vi "getDecay.vi"(8 "error in (no error)":errorcluster, 11 "LaguerreDeconClass in":refnum<class "LaguerreDeconEngineClass.lvclass">) -> (0 "error out":errorcluster, 2 "Decay":dbl[](array[numeric]), 3 "LaguerreDeconClass out":refnum<class "LaguerreDeconEngineClass.lvclass">)   [LabVIEW 2020, in "LaguerreDeconEngineClass.lvclass"]
uses:
  LaguerreDeconEngineClass.lvclass
  LaguerreDeconEngineClass.lvclass/LaguerreDeconEngineClass.ctl
  <vilib>/Analysis/baseanly.llb/A x Vector.vi
  <vilib>/Analysis/NI_AALBase.lvlib
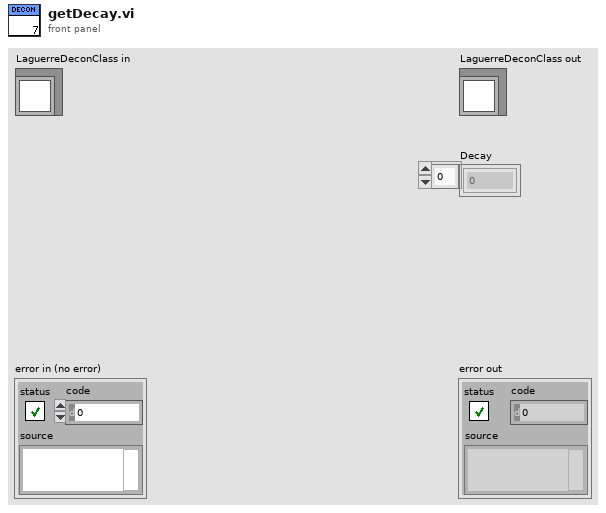
[diagram p1: front panel]
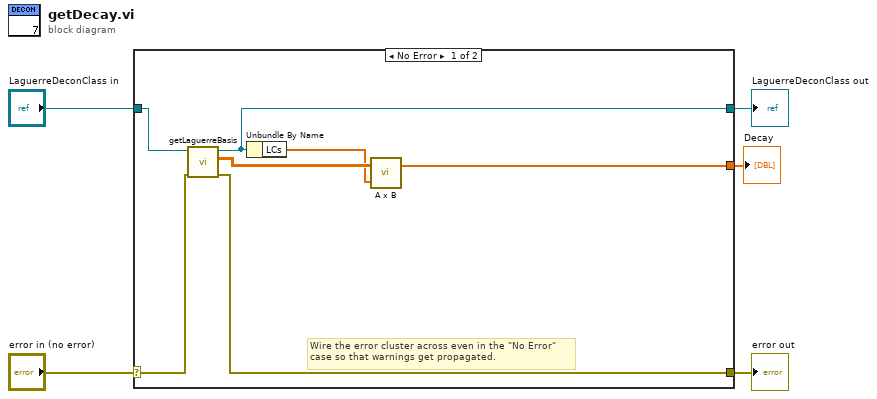
[diagram p0: block diagram]
diagram:
  n1 = case shown="No Error" "error in (no error)" {
    selector: "error in (no error)" -> [w9 w14]
    tunnel: [w8 w14] -> w4
    tunnel: [w6 w13] -> w2
    tunnel: "LaguerreDeconClass in" -> [w12 w13]
    tunnel: [w7 _] -> w1
    frame No Error {
      # "Wire the error cluster across even in the \"No Error\"\ncase so that warnings get propagated."
      n2 = call "getLaguerreBasis.vi"("error in (no error)"=w9, "LaguerreDeconClass in"=w12) -> ("error out"=w8:errorcluster, "laguerreBasis"=w11:dbl[][], "LaguerreDeconClass out"=w6:refnum<class "LaguerreDeconEngineClass.lvclass">)  [unwired: 7 in]
      n3 = Unbundle By Name(w6) -> ("LCs"=w10:dbl[])
      n4 = call-poly <vilib>:"A x B.vi"("Vector"=w10, "A"=w11) -> ("A x Vector"=w7:dbl[])  [unwired: 1 out]
    }
    frame Error {
    }
  }
  "error out" <- w4
  "LaguerreDeconClass out" <- w2
  "Decay" <- w1
